vi "Read Data.vi"(8 "AI Rate":dbl=10000.0 format="%.2f", 9 "AI Buffer Size (s)":i32=10, 10 "AI Block Size":i32=5000, 11 "AI task":refnum<k21>[](array[refnum])=["", ""]) -> (1 "Backlog":u8(slide) scale=0.0..100.0, 2 "Input Signals":dbl[][](array[numeric]), 3 "Input Signals":waveform(dbl)[](array[waveform]))   [LabVIEW 2013]
uses:
  <vilib>/DAQmx/read.llb/DAQmx Read (Analog 1D Wfm NChan NSamp).vi
  <vilib>/DAQmx/miscellaneous.llb/DAQmx Fill In Error Info.vi
  <vilib>/DAQmx/read.llb/DAQmx Read (Analog 2D DBL NChan NSamp).vi
  <resource>/objmgr/daqmx.rc
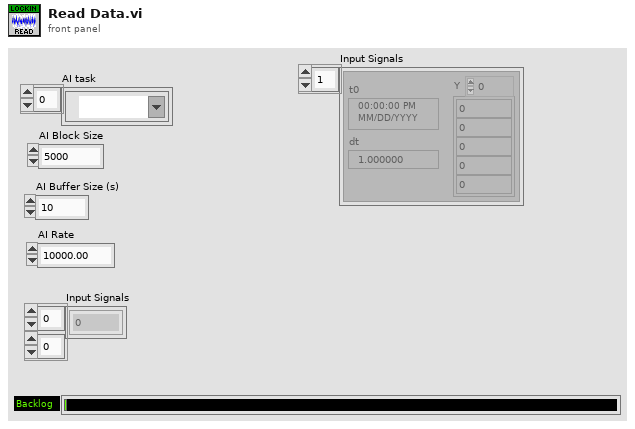
[diagram p1: front panel]
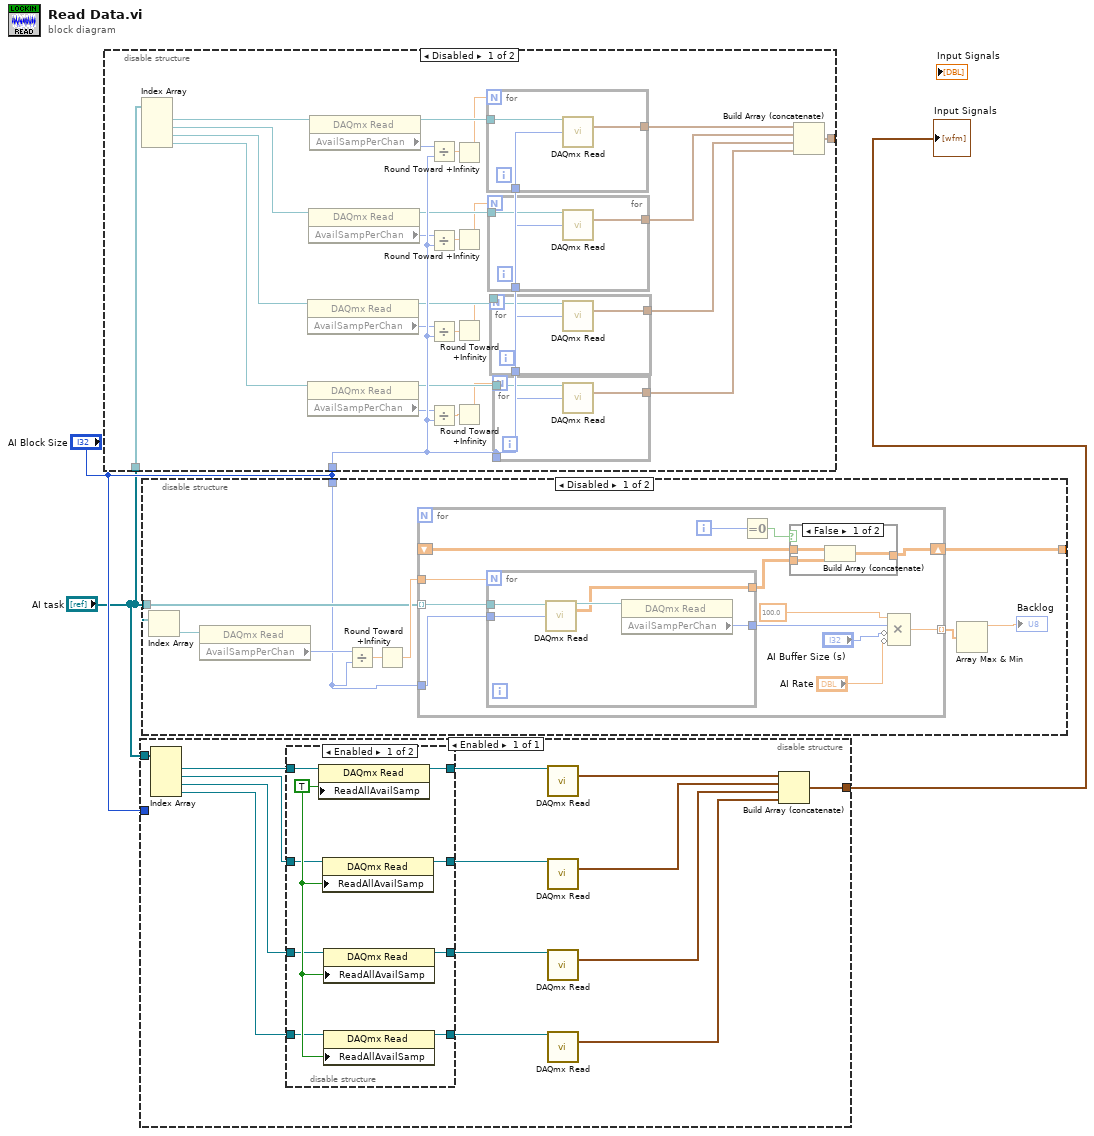
[diagram p0: block diagram]
diagram:
  n1 = disable-structure shown="Disabled" {
    disable-tunnel: "AI task" -> [w30 _]
    disable-tunnel: "AI Block Size" -> [w29 _]
    disable-tunnel: [w4 _] -> _
    frame Disabled {
      n2 = Index Array(array=w30) -> (element #1=w21:refnum<k21>, element #2=w22:refnum<k21>, element #3=w23:refnum<k21>, element #4=w24:refnum<k21>)  [unwired: 4 in]
      n3 = property class="DAQmx Read"(reference=w23) -> (reference out=w18:refnum<k21>, "AvailSampPerChan"=w14:u32)  [unwired: 1 in, 1 out]
      n4 = property class="DAQmx Read"(reference=w24) -> (reference out=w17:refnum<k21>, "AvailSampPerChan"=w15:u32)  [unwired: 1 in, 1 out]
      n5 = property class="DAQmx Read"(reference=w22) -> (reference out=w19:refnum<k21>, "AvailSampPerChan"=w13:u32)  [unwired: 1 in, 1 out]
      n6 = property class="DAQmx Read"(reference=w21) -> (reference out=w20:refnum<k21>, "AvailSampPerChan"=w16:u32)  [unwired: 1 in, 1 out]
      n7 = Divide(x=w16, y=w29) -> (x/y=w12:dbl)
      n8 = Divide(x=w13, y=w29) -> (x/y=w11:dbl)
      n9 = Divide(x=w14, y=w29) -> (x/y=w10:dbl)
      n10 = Divide(x=w15, y=w29) -> (x/y=w9:dbl)
      n11 = Round Toward +Infinity(x=w12) -> (ceil(x): smallest int >= x=w5:dbl)
      n12 = Round Toward +Infinity(x=w11) -> (ceil(x): smallest int >= x=w6:dbl)
      n13 = Round Toward +Infinity(x=w10) -> (ceil(x): smallest int >= x=w7:dbl)
      n14 = Round Toward +Infinity(x=w9) -> (ceil(x): smallest int >= x=w8:dbl)
      n15 = for {
        N: w5 -> [_]
        tunnel: [w42] -> w25
        tunnel: w20 -> [w41]
        tunnel: w29 -> [w40]
        n16 = call-poly <vilib>:"DAQmx Read.vi"("task/channels in"=w41, "number of samples per channel"=w40) -> ("data"=w42:waveform(dbl)[])  [unwired: 11 in, 2 out]
      }
      n17 = for {
        N: w6 -> [_]
        tunnel: [w39] -> w26
        tunnel: w19 -> [w38]
        tunnel: w29 -> [w37]
        n18 = call-poly <vilib>:"DAQmx Read.vi"("task/channels in"=w38, "number of samples per channel"=w37) -> ("data"=w39:waveform(dbl)[])  [unwired: 11 in, 2 out]
      }
      n19 = for {
        N: w7 -> [_]
        tunnel: [w36] -> w27
        tunnel: w18 -> [w35]
        tunnel: w29 -> [w34]
        n20 = call-poly <vilib>:"DAQmx Read.vi"("task/channels in"=w35, "number of samples per channel"=w34) -> ("data"=w36:waveform(dbl)[])  [unwired: 11 in, 2 out]
      }
      n21 = for {
        N: w8 -> [_]
        tunnel: [w33] -> w28
        tunnel: w17 -> [w32]
        tunnel: w29 -> [w31]
        n22 = call-poly <vilib>:"DAQmx Read.vi"("task/channels in"=w32, "number of samples per channel"=w31) -> ("data"=w33:waveform(dbl)[])  [unwired: 11 in, 2 out]
      }
      n23 = Build Array (concatenate)(w25, w26, w27, w28) -> (w4:waveform(dbl)[])
    }
    frame Enabled {
    }
  }
  n24 = disable-structure shown="Enabled" {
    disable-tunnel: "AI task" -> [w56]
    disable-tunnel: "AI Block Size" -> [_]
    disable-tunnel: [w43] -> w2
    frame Enabled {
      n25 = Index Array(array=w56) -> (element #1=w55:refnum<k21>, element #2=w50:refnum<k21>, element #3=w49:refnum<k21>, element #4=w48:refnum<k21>)  [unwired: 4 in]
      n26 = disable-structure shown="Enabled" {
        disable-tunnel: w55 -> [w65 w69]
        disable-tunnel: [w64 w69] -> w54
        disable-tunnel: [w63 w66] -> w53
        disable-tunnel: [w62 w67] -> w52
        disable-tunnel: [w61 w68] -> w51
        disable-tunnel: w50 -> [w59 w68]
        disable-tunnel: w49 -> [w58 w67]
        disable-tunnel: w48 -> [w57 w66]
        frame Enabled {
          w60 = TRUE ("ReadAllAvailSamp")
          n27 = property class="DAQmx Read"(reference=w65, "ReadAllAvailSamp"=w60) -> (reference out=w64:refnum<k21>)  [unwired: 1 in, 1 out]
          n28 = property class="DAQmx Read"(reference=w59, "ReadAllAvailSamp"=w60) -> (reference out=w61:refnum<k21>)  [unwired: 1 in, 1 out]
          n29 = property class="DAQmx Read"(reference=w58, "ReadAllAvailSamp"=w60) -> (reference out=w62:refnum<k21>)  [unwired: 1 in, 1 out]
          n30 = property class="DAQmx Read"(reference=w57, "ReadAllAvailSamp"=w60) -> (reference out=w63:refnum<k21>)  [unwired: 1 in, 1 out]
        }
        frame Disabled {
        }
      }
      n31 = call-poly <vilib>:"DAQmx Read.vi"("task/channels in"=w54) -> ("data"=w47:waveform(dbl)[])  [unwired: 12 in, 2 out]
      n32 = call-poly <vilib>:"DAQmx Read.vi"("task/channels in"=w51) -> ("data"=w46:waveform(dbl)[])  [unwired: 12 in, 2 out]
      n33 = call-poly <vilib>:"DAQmx Read.vi"("task/channels in"=w52) -> ("data"=w45:waveform(dbl)[])  [unwired: 12 in, 2 out]
      n34 = call-poly <vilib>:"DAQmx Read.vi"("task/channels in"=w53) -> ("data"=w44:waveform(dbl)[])  [unwired: 12 in, 2 out]
      n35 = Build Array (concatenate)(w47, w46, w45, w44) -> (w43:waveform(dbl)[])
    }
  }
  "Input Signals" <- w2
  n36 = disable-structure shown="Disabled" {
    disable-tunnel: [w72 _] -> _
    disable-tunnel: "AI task" -> [w71 _]
    disable-tunnel: "AI Block Size" -> [w70 _]
    frame Disabled {
      n37 = Index Array(array=w71) -> (element=w76:refnum<k21>)  [unwired: 1 in]
      n38 = property class="DAQmx Read"(reference=w76) -> ("AvailSampPerChan"=w75:u32)  [unwired: 1 in, 2 out]
      n39 = Divide(x=w75, y=w70) -> (x/y=w74:dbl)
      n40 = Round Toward +Infinity(x=w74) -> (ceil(x): smallest int >= x=w73:dbl)
      n41 = for {
        tunnel: w71 -> [w83] mode=indexing
        tunnel: [w89] -> w78 mode=indexing
        shift-right: [w84] -> w72
        shift-left: _ -> [w86]
        tunnel: w73 -> [w82]
        tunnel: w70 -> [w81]
        i -> [w87]
        n42 = for {
          N: w82 -> [_]
          tunnel: [w99] -> w85
          tunnel: [w98] -> w91
          tunnel: w83 -> [w97]
          tunnel: w81 -> [w96]
          n43 = call-poly <vilib>:"DAQmx Read.vi"("task/channels in"=w97, "number of samples per channel"=w96) -> ("task out"=w100:refnum<k21>, "data"=w99:dbl[][])  [unwired: 11 in, 1 out]
          n44 = property class="DAQmx Read"(reference=w100) -> ("AvailSampPerChan"=w98:u32)  [unwired: 1 in, 2 out]
        }
        n45 = Equal To 0?(x=w87) -> (x = 0?=w88:bool)
        n46 = case shown="False" w88 {
          tunnel: w86 -> [w92 _]
          tunnel: w85 -> [w94 w95]
          tunnel: [w93 w95] -> w84
          frame False {
            n47 = Build Array (concatenate)(w92, w94) -> (w93:dbl[][])
          }
          frame True {
          }
        }
        n48 = Compound Arithmetic op=MULTIPLY(100.0 ("value"), w91, invert "AI Buffer Size (s)", invert "AI Rate") -> (w89:dbl)
      }
      n49 = Array Max & Min(array=w78) -> (max value=→"Backlog":dbl)  [unwired: 3 out]
    }
    frame Enabled {
    }
  }
